vi "SimulateAcquisitionTest.vi"() -> ()   [LabVIEW 2015]
uses:
  <vilib>/vision/NI_Vision_Development_Module.lvlib
panel:
  in  "stop":bool
  out "Image":T1(plugin-control)
  out "Centroid":cluster{"X Centroid":sgl, "Y Centroid":sgl} {"Y Centroid" format="%.2f"; "X Centroid" format="%.2f"}
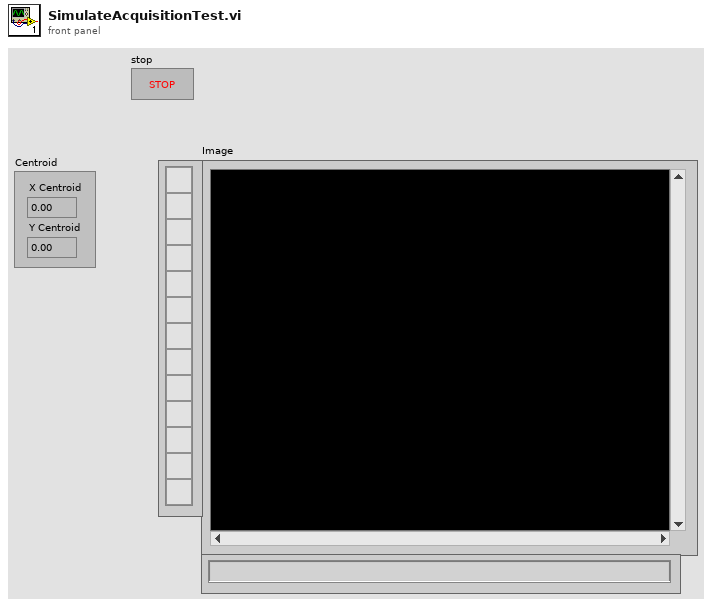
[diagram p1: front panel]
types:
  T1 = typedef "IMAQ Image.ctl" = refnum<image>
  T2 = typedef "Image Type" = u32
  T3 = cluster{"Global Rectangle":i32[], "Contours":cluster{"Contour Type":u32, "ROI Type":u32, "Points":i32[]}[]}
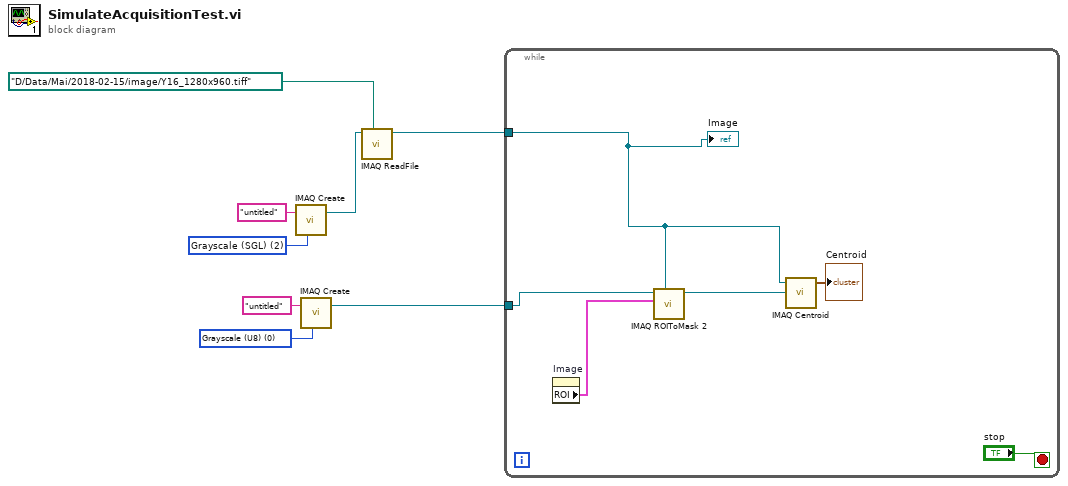
[diagram p0: block diagram]
diagram:
  w6 = T2 0 items=["Grayscale (U8)", "Grayscale (I16)", "Grayscale (SGL)", "Complex (CSG)", "RGB (U32)", "HSL (U32)", "RGB (U64)", "Grayscale (U16)"] ("Image Type")
  w7 = T2 2 items=["Grayscale (U8)", "Grayscale (I16)", "Grayscale (SGL)", "Complex (CSG)", "RGB (U32)", "HSL (U32)", "RGB (U64)", "Grayscale (U16)"] ("Image Type")
  n1 = call "IMAQ Create"("Image Name"="untitled", "Image Type"=w7) -> ("New Image"=w2:T1)  [unwired: 3 in, 1 out]
  n2 = call "IMAQ Create"("Image Name"="untitled", "Image Type"=w6) -> ("New Image"=w8:T1)  [unwired: 3 in, 1 out]
  n3 = call "IMAQ ReadFile"("File Path"=path "D:/Data/Mai/2018-02-15/image/Y16_1280x960.tiff", "Image"=w2) -> ("Image Out"=w1:T1)  [unwired: 5 in, 4 out]
  n4 = while {
    tunnel: w8 -> [w13]
    tunnel: w1 -> [w11]
    stop <- "stop" stop-if-true
    n5 = property on="Image" class="ImageControl"() -> ("ROI"=w9:T3)  [unwired: 2 in, 2 out]
    n6 = call "IMAQ ROIToMask 2"("Image Model"=w11, "ROI Descriptor"=w9, "Image"=w13) -> ("Image Out"=w14:T1)  [unwired: 6 in, 2 out]
    n7 = call "IMAQ Centroid"("Image Mask"=w14, "Image"=w11) -> ("Centroid"=→"Centroid":cluster{"X Centroid":sgl, "Y Centroid":sgl})  [unwired: 2 in, 1 out]
    "Image" <- w11
  }
